vi "loop-for.vi"() -> ()   [LabVIEW 2020, in "Library 1.lvlib"]
uses:
  Libs/Library 1.lvlib
panel:
  out "s? t:f":dbl[](array[numeric])
  in  "Boolean 2":bool
  out "String":string
  out "Boolean":bool
  in  "N VALUE":dbl
  out "Slide 2":dbl(slide) scale=0.0..100.0
  out "1 VALUE":i32
  in  "ARRAY 2 -1":dbl
  in  "ARRAY 1-1":dbl
  in  "ARRAY 2-2":dbl
  in  "ARRAY 1 -0":dbl
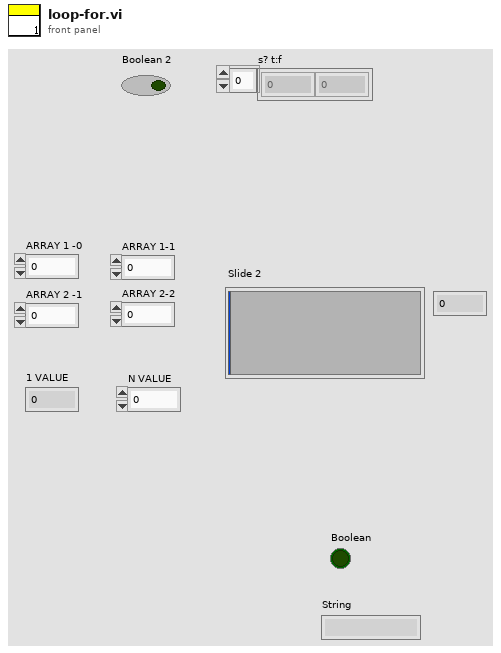
[diagram p1: front panel]
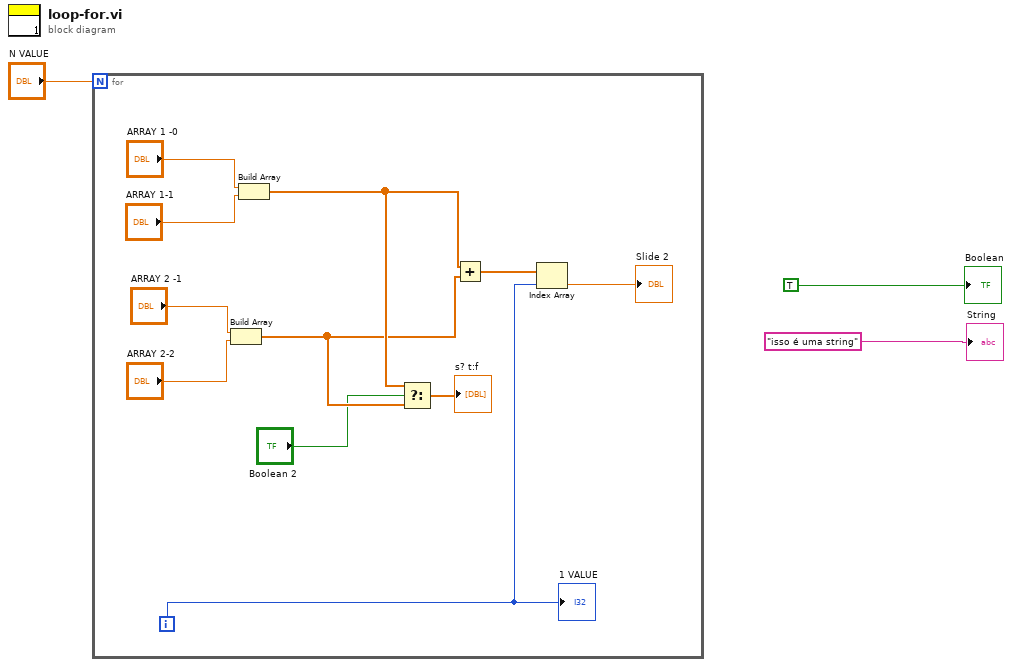
[diagram p0: block diagram]
diagram:
  n1 = for {
    N: "N VALUE" -> [_]
    i -> [w9]
    n2 = Build Array("ARRAY 2 -1", "ARRAY 2-2") -> (w6:dbl[])
    n3 = Build Array("ARRAY 1 -0", "ARRAY 1-1") -> (w7:dbl[])
    n4 = Select(t=w7, s="Boolean 2", f=w6) -> (s? t:f=→"s? t:f":dbl[])
    n5 = Add(x=w7, y=w6) -> (x+y=w10:dbl[])
    n6 = Index Array(array=w10, index=w9) -> (element=→"Slide 2":dbl)
    "1 VALUE" <- w9
  }
  "Boolean" <- TRUE
  "String" <- "isso é uma string"
